vi "Add Section.vi"(7 "GUID (Default Section)":string="03D3BB89-1485-13A6-56005DE6430FF8B7", 8 "error in (no error)":errorcluster, 10 "Section Name":string, 11 "Item Ref in":T1 format="%.0x") -> (0 "error out":errorcluster, 2 "Status Section Ptr":T1 format="%.0x", 3 "Item Ref out":T1 format="%.0x")   [LabVIEW 2017, in "DSF System Explorer.lvlib"]
uses:
  DSF System Explorer.lvlib
  <vilib>/NI Veristand/Custom Device API/Custom Device Item Ref.ctl
  <vilib>/NI Veristand/Custom Device API/Custom Device API.lvlib
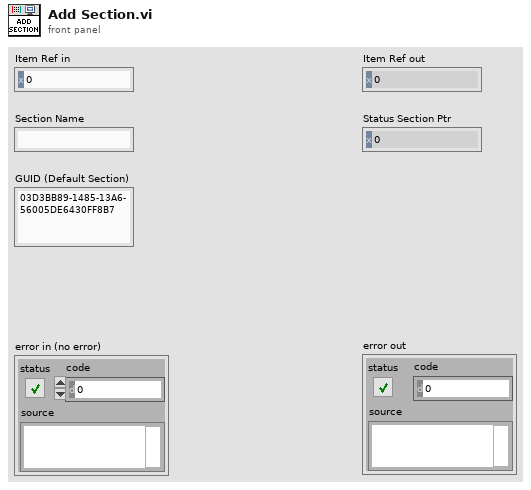
[diagram p1: front panel]
types:
  T1 = typedef "Custom Device API.lvlib/Custom Device Item Ref.ctl" = u64
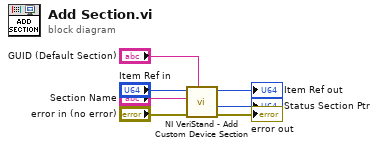
[diagram p0: block diagram]
diagram:
  n1 = call <vilib>:"NI VeriStand - Add Custom Device Section.vi"("GUID (Default Section)"="GUID (Default Section)", "error in (no error)"="error in (no error)", "Section Name"="Section Name", "Parent Ref in"="Item Ref in") -> ("error out"=→"error out":errorcluster, "Section Ptr"=→"Status Section Ptr":T1, "Parent Ref out"=→"Item Ref out":T1)  [unwired: 4 in, 1 out]
